vi "未命名 2.vi"() -> ()   [LabVIEW 2012]
panel:
  out "强度图表":dbl[][](graph)
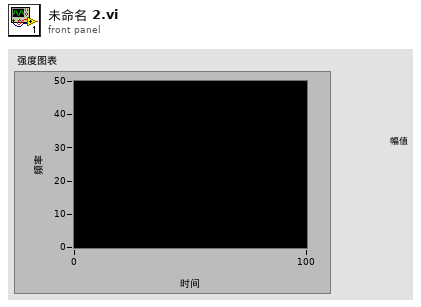
[diagram p1: front panel]
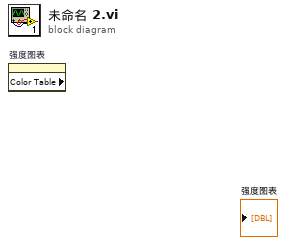
[diagram p0: block diagram]
diagram:
  n1 = property on="强度图表" class="IntChart (严格)" props=["Color Table"]() -> ()  [unwired: 2 in, 3 out]
